vi "VoltageToAngleValve.vi"(11 "Voltage":dbl) -> (3 "Angle":dbl)   [LabVIEW 2022 SP3]
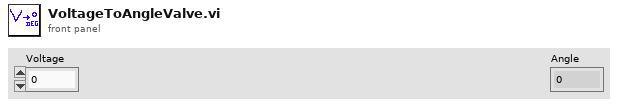
[diagram p1: front panel]
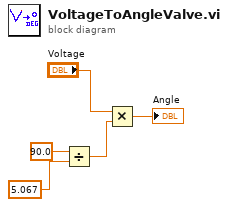
[diagram p0: block diagram]
diagram:
  n1 = Divide(x=90.0, y=5.067) -> (x/y=w3:dbl)
  n2 = Multiply(x="Voltage", y=w3) -> (x*y=→"Angle":dbl)
